vi "APS ptp all.vi"(0 "Axis_ID":i32, 1 "Vm":dbl, 2 "Acc":dbl, 3 "SFac":dbl, 5 "Option":i32, 7 "Position":dbl, 9 "Vs":dbl, 11 "error in (no error)":errorcluster caption="错误输入（无错误）", 12 "Ve":dbl, 13 "Dec":dbl, 14 "Wait":cluster{"h_event":u32, "i32_ret":i32}) -> (4 "Wait out":cluster{"h_event":u32, "i32_ret":i32}, 6 "function return":i32, 15 "error out":errorcluster caption="错误输出")   [LabVIEW 2011, in "APS168.lvlib"]
doc: "I32 FNTYPE APS_ptp_all( I32 Axis_ID, I32 Option, F64 Position, F64 Vs, F64 Vm, F64 Ve, F64 Acc, F64 Dec, F64 SFac, ASYNCALL *Wait);"
uses:
  APS168.lvlib
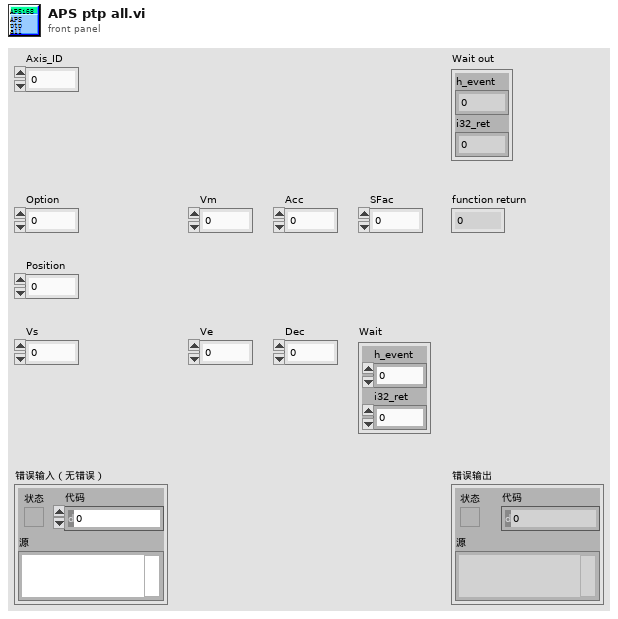
[diagram p1: front panel]
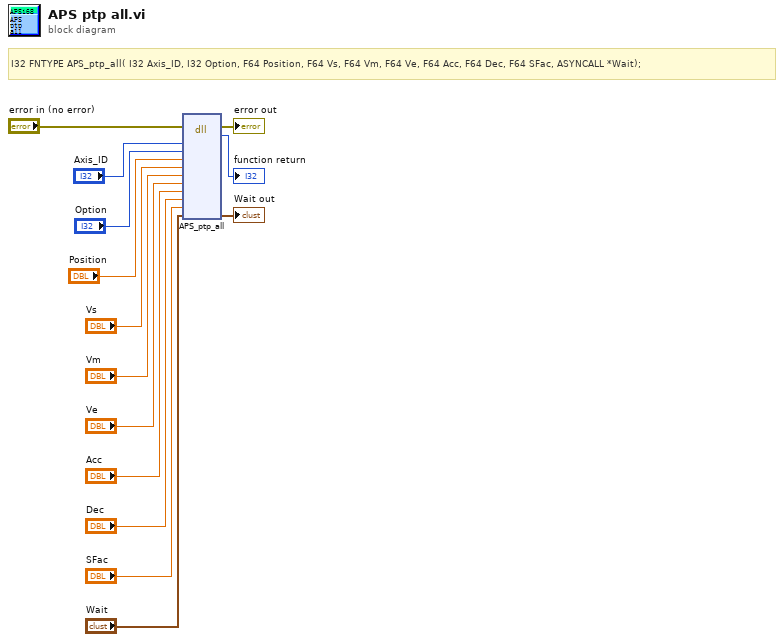
[diagram p0: block diagram]
diagram:
  # "I32 FNTYPE APS_ptp_all( I32 Axis_ID, I32 Option, F64 Position, F64 Vs,\tF64 Vm, F64\tVe, F64 Acc,\tF64 Dec, F64 SFac, ASYNCALL *Wait);"
  n1 = dll-call lib="PTH1Labs E软件ADLINK 204CAPS_1_7_1_LIB line 连续运动204APS168.*" fn="APS_ptp_all"(error in="error in (no error)", "Axis_ID"="Axis_ID", "Option"="Option", "Position"="Position", "Vs"="Vs", "Vm"="Vm", "Ve"="Ve", "Acc"="Acc", "Dec"="Dec", "SFac"="SFac", "Wait"="Wait") -> (error out=→"error out":errorcluster, →"function return":i32, "Wait"=→"Wait out":cluster{"h_event":u32, "i32_ret":i32})  [unwired: 11 in, 1 out]
